vi "Xbox Event Structure.vi"() -> ()   [LabVIEW 2011, in "LVH-Xbox-One-Controller.lvlib"]
doc: "This VI places an Xbox Controller Open, Event structure with all Xbox Controller Events pre populated and an Xbox Controller close VI."
uses:
  LVH-Xbox-One-Controller.lvlib
panel:
  in  "Device Index":i32=4
  in  "Stop Button":bool
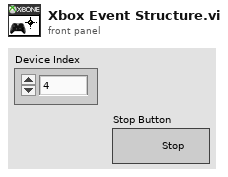
[diagram p1: front panel]
types:
  T1 = typedef "LVH-Xbox-One-Controller.lvlib/Xbox One Controller Ref.ctl" = cluster{"Controller Ref":refnum<k1>, "Event Refnum":refnum<event-registration>, "Worker Ref":refnum<vi>}
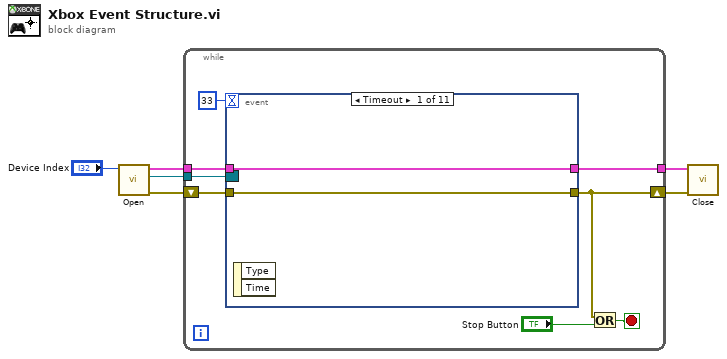
[diagram p0: block diagram]
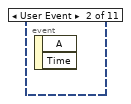
[diagram p2: hidden frame]
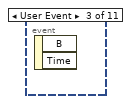
[diagram p3: hidden frame]
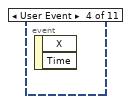
[diagram p4: hidden frame]
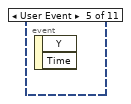
[diagram p5: hidden frame]
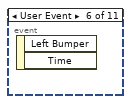
[diagram p6: hidden frame]
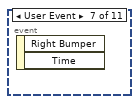
[diagram p7: hidden frame]
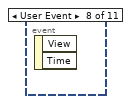
[diagram p8: hidden frame]
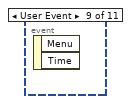
[diagram p9: hidden frame]
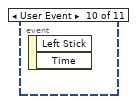
[diagram p10: hidden frame]
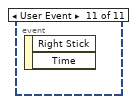
[diagram p11: hidden frame]
diagram:
  n1 = call "Open.vi"("Device Index"="Device Index") -> ("Error Out"=w4:errorcluster, "Event Refnum"=w5:refnum<event-registration>, "Xbox One Controller Ref"=w6:T1)  [unwired: 8 in]
  n2 = while {
    tunnel: w5 -> [w7]
    shift-right: [w10] -> w3
    shift-left: w4 -> [w13]
    tunnel: w6 -> [w14]
    tunnel: [w9] -> w2
    stop <- w12 stop-if-true
    n3 = event shown="[0] Timeout" {
      selector: w7 -> [_ _ _ _ _ _ _ _ _ _ _]
      dyn-events: _ -> [_ _ _ _ _ _ _ _ _ _ _]
      timeout: 33 -> [_ _ _ _ _ _ _ _ _ _ _]
      tunnel: w14 -> [w16 _ _ _ _ _ _ _ _ _ _]
      tunnel: w13 -> [w15 _ _ _ _ _ _ _ _ _ _]
      tunnel: [w15 _ _ _ _ _ _ _ _ _ _] -> w10
      tunnel: [w16 _ _ _ _ _ _ _ _ _ _] -> w9
      event Timeout {
        n4 = event-data() -> ()  [unwired: 1 in, 2 out]
      }
      event User Event {
        n5 = event-data() -> ()  [unwired: 1 in, 2 out]
      }
      event User Event {
        n6 = event-data() -> ()  [unwired: 1 in, 2 out]
      }
      event User Event {
        n7 = event-data() -> ()  [unwired: 1 in, 2 out]
      }
      event User Event {
        n8 = event-data() -> ()  [unwired: 1 in, 2 out]
      }
      event User Event {
        n9 = event-data() -> ()  [unwired: 1 in, 2 out]
      }
      event User Event {
        n10 = event-data() -> ()  [unwired: 1 in, 2 out]
      }
      event User Event {
        n11 = event-data() -> ()  [unwired: 1 in, 2 out]
      }
      event User Event {
        n12 = event-data() -> ()  [unwired: 1 in, 2 out]
      }
      event User Event {
        n13 = event-data() -> ()  [unwired: 1 in, 2 out]
      }
      event User Event {
        n14 = event-data() -> ()  [unwired: 1 in, 2 out]
      }
    }
    n15 = Or(x=w10, y="Stop Button") -> (x .or. y?=w12:bool)
  }
  n16 = call "Close.vi"("Error In"=w3, "Xbox One Controller Ref"=w2) -> ()  [unwired: 9 in, 1 out]
